vi "Actor Core.vi"(8 "error in":errorcluster, 11 "File Provider in":refnum<class "File Provider.lvclass">) -> (0 "error out":errorcluster, 3 "Actor out":refnum<class "Actor.lvclass">)   [LabVIEW 2024, in "File Provider.lvlib" / "File Provider.lvclass"]
doc: "(<B>Filename</B>: Actor Framework.lvlib:Actor.lvclass:Actor Core.vi)\n\nReceives messages to the actor, reacts to them, and initiates any error handling that may shut the actor down.\n\nDescendant classes may override this VI to append parallel tasks for the actor to complete while it handles messages. Overrides use the Call Parent Class Method node."
uses:
  File Provider.lvclass
  File Provider.lvclass/File Provider.ctl
  <vilib>/MGI/Panel Manager/Panel Actor/Panel Actor/Panel Actor.lvclass
  File Provider Messages/Read Series CFG Msg/Read Series CFG Msg.lvclass
  File Provider Messages/Read Virt Instr CFG Msg/Read Virt Instr CFG Msg.lvclass
  File Provider Messages/Read and Add Instr CFGs Msg/Read and Add Instr CFGs Msg.lvclass
  IConfiguration UI Actor/IConfiguration UI Actor Messages/Set Virt Instr CFG Msg/Set Virt Instr CFG Msg.lvclass
  IConfiguration UI Actor/IConfiguration UI Actor Messages/Add Instr CFG Msg/Add Instr CFG Msg.lvclass
  IConfiguration UI Actor/IConfiguration UI Actor Messages/Set Series CFG Msg/Set Series CFG Msg.lvclass
  <vilib>/ActorFramework/Actor/Actor.lvclass
panel:
  in  "Refresh Series CFG":bool
  in  "Refresh Virt Instrs CFG":bool
  out "Series CFG":string
  out "Virt Instrs CFG":string
  in  "Clear Instr CFGs Button":bool
  in  "Open Instr CFGs":bool
  in  "Load":bool
  out "Instrument CFGs":string[](array[string])
  in  "Series CFG Path":path
  in  "Virt Instrs CFG Path":path
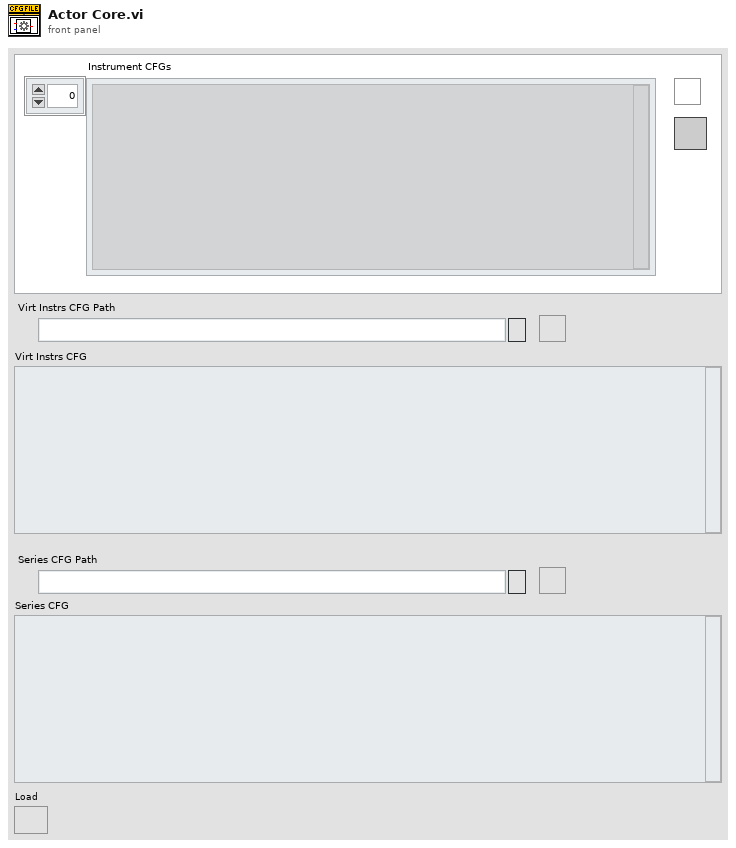
[diagram p1: front panel]
types:
  T1 = enum32{"existing file", "new file", "new or existing file", "existing dir", "new dir", "new or existing dir", "existing file (use LLBs)", "new file (use LLBs)", "new or existing file (use LLBs)", "new or existing file or directory (use LLBs)", "existing dir (use LLBs)", "new dir (use LLBs)", "new or existing dir (use LLBs)", "existing file or dir", "new file or dir", "new or existing file or dir", "existing file or dir (use LLBs)", "new file or dir (use LLBs)", "multi-select", "multi-select (use LLBs)"}
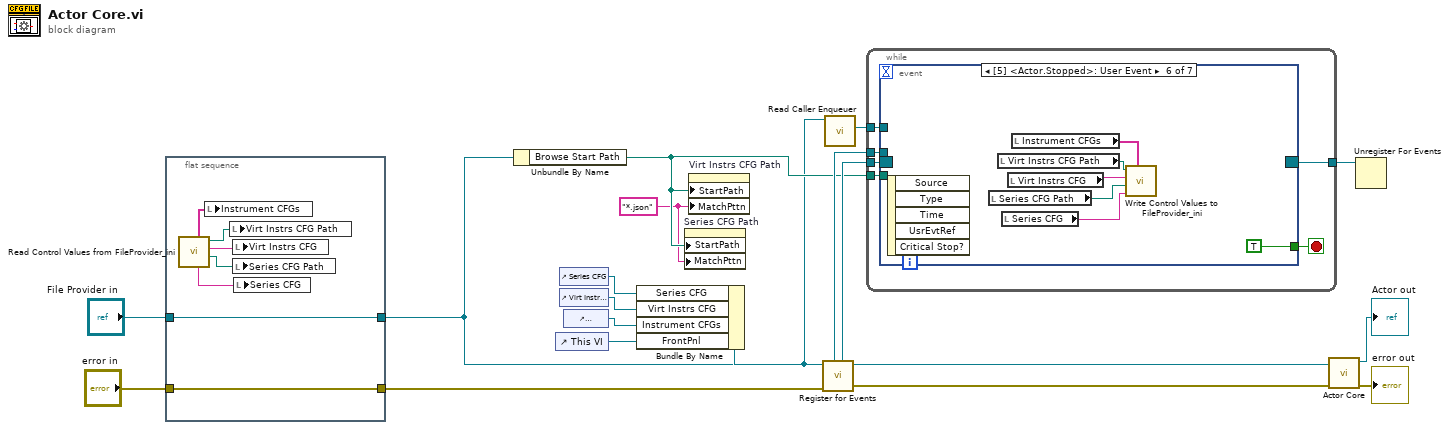
[diagram p0: block diagram]
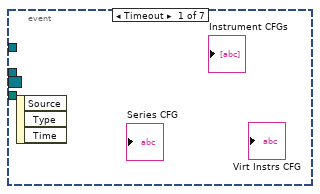
[diagram p2: hidden frame]
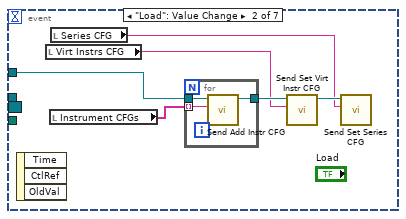
[diagram p3: hidden frame]
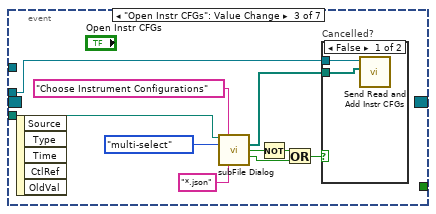
[diagram p4: hidden frame]
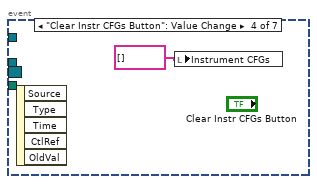
[diagram p6: hidden frame]
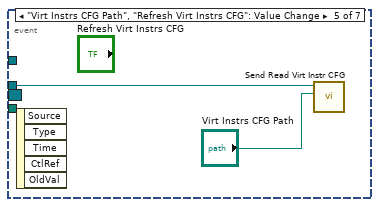
[diagram p7: hidden frame]
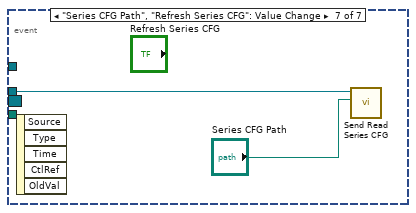
[diagram p8: hidden frame]
diagram:
  w5 = "*.json" ("Browse Options:Match Pattern")
  n1 = flat-sequence {
    tunnel: "File Provider in" -> [w26]
    tunnel: [w26] -> w3
    tunnel: "error in" -> [w25]
    tunnel: [w25] -> w1
    frame #0 {
      n2 = call "Read Control Values from FileProvider_ini.vi"() -> ("Series CFG Path Value"=w21:path, "Virt Instrs CFG Value"=w22:string, "Virt Instrs CFG Path Value"=w23:path, "Series CFG Value"=w20:string, "Instrument CFGs"=w24:string[])  [unwired: 6 in, 1 out]
      n3 = local write "Instrument CFGs"(w24) -> ()
      n4 = local write "Virt Instrs CFG Path"(w23) -> ()
      n5 = local write "Virt Instrs CFG"(w22) -> ()
      n6 = local write "Series CFG Path"(w21) -> ()
      n7 = local write "Series CFG"(w20) -> ()
    }
  }
  n8 = Unbundle By Name(w3) -> ("Browse Start Path"=w12:path)
  n9 = control-ref of="This VI"() -> (w16:refnum<vi>)
  n10 = control-ref of="Series CFG"() -> (w9:refnum<vi>)
  n11 = control-ref of="Virt Instrs CFG"() -> (w8:refnum<vi>)
  n12 = control-ref of="Instrument CFGs"() -> (w11:refnum<vi>)
  n13 = Bundle By Name(cluster=w3, "Series CFG"=w9, "Virt Instrs CFG"=w8, "Instrument CFGs"=w11, "FrontPnl"=w16) -> (w6:refnum<class "File Provider.lvclass">)
  n14 = property on="Series CFG Path" class="Path"("StartPath"=w12, "MatchPttn"=w5) -> ()  [unwired: 2 in, 2 out]
  n15 = property on="Virt Instrs CFG Path" class="Path"("StartPath"=w12, "MatchPttn"=w5) -> ()  [unwired: 2 in, 2 out]
  n16 = call <vilib>:"Register for Events.vi"("Error In"=w1, "Panel Actor in"=w6) -> ("Error Out"=w17:errorcluster, "Panel Actor out"=w13:refnum<class "File Provider.lvclass">, "Pnl Actor"=w15:refnum<event-registration>, "Self Enqueuer"=w14:refnum<class "Message Enqueuer.lvclass">)  [unwired: 6 in]
  n17 = call <vilib>:"Read Caller Enqueuer.vi"("Actor"=w6) -> ("Caller Enqueuer"=w7:refnum<class "Message Enqueuer.lvclass">)  [unwired: 10 in]
  n18 = while {
    tunnel: w15 -> [w32]
    tunnel: w14 -> [w31]
    tunnel: w12 -> [w29]
    tunnel: [w28] -> w10
    tunnel: w7 -> [w27]
    stop <- w30 stop-if-true
    n19 = event shown="[5] <Actor.Stopped>: User Event" {
      selector: w32 -> [_ _ _ _ _ _ _]
      dyn-events: [_ _ _ _ _ _ _] -> w28
      timeout: _ -> [_ _ _ _ _ _ _]
      tunnel: w31 -> [_ _ w51 _ w56 _ w64]
      tunnel: [_ _ _ _ _ TRUE _] -> w30
      tunnel: w29 -> [_ _ w46 _ _ _ _]
      tunnel: w27 -> [_ w33 _ _ _ _ _]
      event Timeout {
        n20 = event-data() -> ()  [unwired: 1 in, 3 out]
      }
      event "Load": Value Change {
        n21 = event-data() -> ()  [unwired: 1 in, 3 out]
        n22 = local read "Virt Instrs CFG"() -> (w35:string)
        n23 = local read "Instrument CFGs"() -> (w36:string[])
        n24 = local read "Series CFG"() -> (w34:string)
        n25 = for {
          tunnel: w36 -> [w41] mode=indexing
          tunnel: w33 -> [w40]
          tunnel: [w39] -> w38
          n26 = call "Send Add Instr CFG.vi"("Instr Configuration"=w41, "Message Enqueuer"=w40) -> ("Message Enqueuer out"=w39:refnum<class "Message Enqueuer.lvclass">)  [unwired: 8 in, 1 out]
        }
        n27 = call "Send Set Virt Instr CFG.vi"("Virt Instr CFG"=w35, "Message Enqueuer"=w38) -> ("Message Enqueuer out"=w37:refnum<class "Message Enqueuer.lvclass">)  [unwired: 8 in, 1 out]
        n28 = call "Send Set Series CFG.vi"("Series CFG"=w34, "Message Enqueuer"=w37) -> ()  [unwired: 8 in, 2 out]
      }
      event "Open Instr CFGs": Value Change {
        n29 = event-data() -> ()  [unwired: 1 in, 5 out]
        n30 = call <vilib>:"subFile Dialog.vi"("start path"=w46, "prompt"="Choose Instrument Configurations", "selection mode"=T1."multi-select", "pattern (all files)"="*.json" ("pattern label")) -> ("selected paths"=w47:path[], "exists"=w44:bool, "cancelled"=w45:bool)  [unwired: 7 in, 2 out]
        n31 = Not(x=w44) -> (.not. x?=w43:bool)
        n32 = Or(x=w43, y=w45) -> (x .or. y?=w42:bool)
        n33 = case "Cancelled?" shown="False" w42 {
          tunnel: w51 -> [w53 _]
          tunnel: w47 -> [w52 _]
          frame False {
            n34 = call "Send Read and Add Instr CFGs.vi"("Instr CFGs"=w52, "Message Enqueuer"=w53) -> ()  [unwired: 8 in, 2 out]
          }
          frame True {
          }
        }
      }
      event "Clear Instr CFGs Button": Value Change {
        n35 = event-data() -> ()  [unwired: 1 in, 5 out]
        n36 = local write "Instrument CFGs"(string[] [] ("Instrument CFGs")) -> ()
      }
      event "Virt Instrs CFG Path", "Refresh Virt Instrs CFG": Value Change {
        n37 = event-data() -> ()  [unwired: 1 in, 5 out]
        n38 = call "Send Read Virt Instr CFG.vi"("Virt Instr CFG"="Virt Instrs CFG Path", "Message Enqueuer"=w56) -> ()  [unwired: 8 in, 2 out]
      }
      event User Event {
        n39 = event-data() -> ()  [unwired: 1 in, 5 out]
        n40 = local read "Series CFG Path"() -> (w58:path)
        n41 = local read "Virt Instrs CFG Path"() -> (w60:path)
        n42 = local read "Series CFG"() -> (w57:string)
        n43 = local read "Virt Instrs CFG"() -> (w59:string)
        n44 = local read "Instrument CFGs"() -> (w61:string[])
        n45 = call "Write Control Values to FileProvider_ini.vi"("Instrument CFGs"=w61, "Series CFG Value"=w57, "Series CFG Path Value"=w58, "Virt Instrs CFG Value"=w59, "Virt Instrs CFG Path Value"=w60) -> ()  [unwired: 6 in, 1 out]
      }
      event "Series CFG Path", "Refresh Series CFG": Value Change {
        n46 = event-data() -> ()  [unwired: 1 in, 5 out]
        n47 = call "Send Read Series CFG.vi"("Series CFG File Path"="Series CFG Path", "Message Enqueuer"=w64) -> ()  [unwired: 8 in, 2 out]
      }
    }
  }
  n48 = call-parent "Actor Core.vi"("error in"=w17, "Panel Actor in"=w13) -> ("error out"=→"error out":errorcluster, "Actor out"=→"Actor out":refnum<class "Actor.lvclass">)  [unwired: 8 in]
  n49 = Unregister For Events(event registration refnum=w10) -> ()  [unwired: 1 in, 1 out]
